vi "类别属性.vi"() -> ()   [LabVIEW 2011]
panel:
  out "x = y?":bool
  out "Application:Kind":T1(ring)
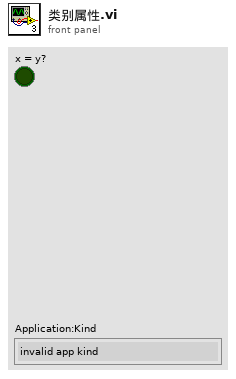
[diagram p1: front panel]
types:
  T1 = enum32{"invalid app kind", "Development System", "Run Time System", "Student Edition", "Embedded LabVIEW", "Evaluation", "Custom"}
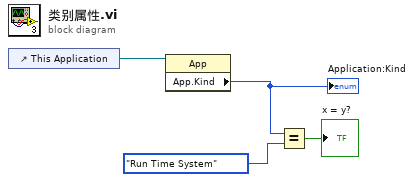
[diagram p0: block diagram]
diagram:
  n1 = control-ref of="This Application"() -> (w4:refnum<vi>)
  n2 = property class="App"(reference=w4) -> ("App.Kind"=w3:T1)  [unwired: 1 in, 2 out]
  "Application:Kind" <- w3
  n3 = Equal?(x=w3, y=T1."Run Time System" ("Application:Kind")) -> (x = y?=→"x = y?":bool)
